vi "Check state.vi"(10 "State":i16, 11 "on state 1":i32) -> (3 "Boolean":bool)   [LabVIEW 2019]
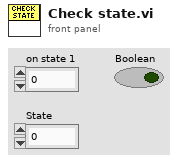
[diagram p1: front panel]
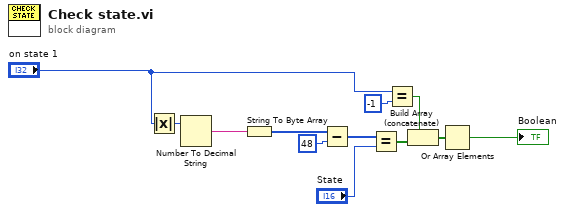
[diagram p0: block diagram]
diagram:
  n1 = Absolute Value(x="on state 1") -> (abs(x)=w10:i32)
  n2 = Number To Decimal String(number=w10) -> (decimal integer string=w12:string)  [unwired: 1 in]
  n3 = String To Byte Array(string=w12) -> (unsigned byte array=w1:u8[])
  n4 = Subtract(x=w1, y=48) -> (x-y=w3:i32[])
  n5 = Equal?(x=w3, y="State") -> (x = y?=w7:bool[])
  n6 = Equal?(x="on state 1", y=-1) -> (x = y?=w8:bool)
  n7 = Build Array (concatenate)(w8, w7) -> (w9:bool[])
  n8 = Or Array Elements(Boolean array=w9) -> (logical OR=→"Boolean":bool)
